vi "Retrieve Element.vi"(8 "error in":errorcluster, 11 "SEQ in":refnum<class "SEQ.lvclass">) -> (0 "error out":errorcluster, 1 "empty?":bool, 2 "STEP.lvclass":refnum<class "STEP.lvclass">, 3 "SEQ out":refnum<class "SEQ.lvclass">)   [LabVIEW 2014, in "Sequence Composition.lvlib" / "SEQ.lvclass"]
doc: "Remove an array element from the top of the sequence stack and return the element removed. If the array is empty (at the end of the sequence) indicate using the <b>empty</b> indicator."
uses:
  SEQ.lvclass
  STEPS/STEP.lvclass
  SEQ.lvclass/SEQ.ctl
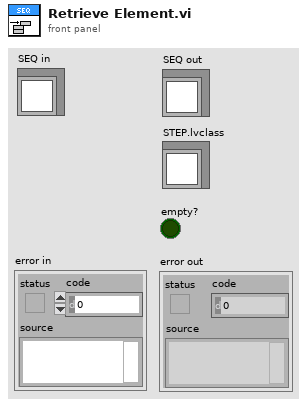
[diagram p1: front panel]
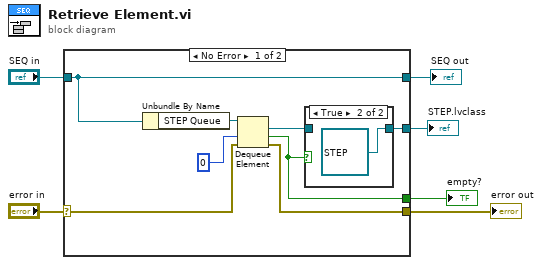
[diagram p0: block diagram]
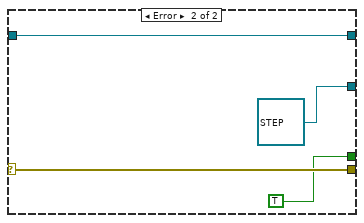
[diagram p3: hidden frame]
diagram:
  n1 = case shown="No Error" "error in" {
    selector: "error in" -> [w8 w20]
    tunnel: [w7 w20] -> w5
    tunnel: [w9 w19] -> w3
    tunnel: "SEQ in" -> [w9 w19]
    tunnel: [w11 refnum<class "STEP.lvclass"> refnum ("STEP.lvclass")] -> w2
    tunnel: [w13 TRUE ("empty?")] -> w1
    frame No Error {
      n2 = Unbundle By Name(w9) -> ("STEP Queue"=w14:refnum<queue>)
      n3 = Dequeue Element(queue=w14, timeout in ms (-1)=0, error in (no error)=w8) -> (element=w12:refnum<class "STEP.lvclass">, timed out?=w13:bool, error out=w7:errorcluster)  [unwired: 1 out]
      n4 = case shown="True" w13 {
        tunnel: [w15 refnum<class "STEP.lvclass"> refnum ("STEP.lvclass")] -> w11
        tunnel: w12 -> [w15 _]
        frame False {
        }
        frame True {
        }
      }
    }
    frame Error {
    }
  }
  "error out" <- w5
  "SEQ out" <- w3
  "STEP.lvclass" <- w2
  "empty?" <- w1
